vi "Close.vi"(8 "error in (no error)":errorcluster, 11 "Modbus slave in":refnum<class "Modbus Slave.lvclass">) -> (0 "error out":errorcluster)   [LabVIEW 2017, in "Modbus Slave.lvclass"]
doc: "Closes and destroys a Modbus slave instance."
uses:
  <vilib>/Modbus/slave/Modbus Slave.lvclass
  <vilib>/Modbus/slave/Modbus Slave.lvclass/Modbus Slave.ctl
  <vilib>/Modbus/subvis/Protocol/Interfaces/Network Slave/Network Slave.lvclass
  <vilib>/Modbus/subvis/Data and Functions/Device Data Model/Device Data Model.lvclass
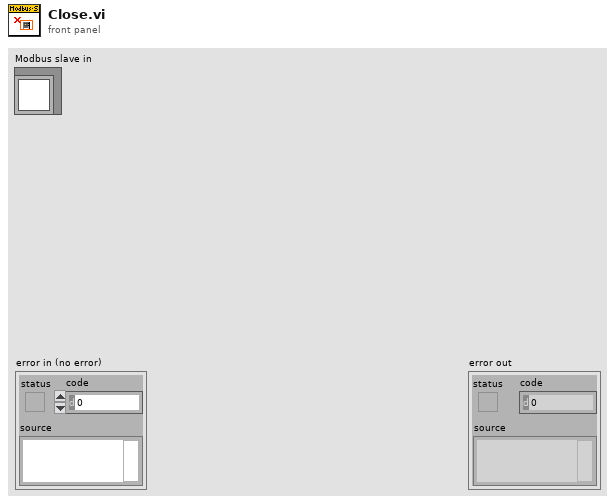
[diagram p1: front panel]
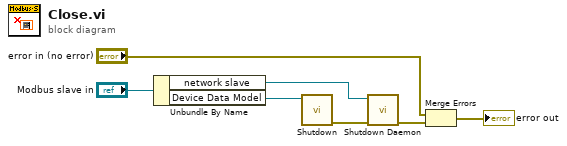
[diagram p0: block diagram]
diagram:
  n1 = Unbundle By Name("Modbus slave in") -> ("network slave"=w5:refnum<class "Network Slave.lvclass">, "Device Data Model"=w4:refnum<class "Device Data Model.lvclass">)
  n2 = call-dynamic "Shutdown.vi"("device data model in"=w4) -> ("error out"=w6:errorcluster)  [unwired: 10 in]
  n3 = call-dynamic "Shutdown Daemon.vi"("error in (no error)"=w6, "network slave in"=w5) -> ("error out"=w2:errorcluster)  [unwired: 9 in]
  n4 = Merge Errors("error in (no error)", w2) -> (→"error out":errorcluster)
